vi "HV Onstate Single.vi"(8 "On/Off":string(combo), 11 "Channel":string) -> (3 "standard output":string)   [LabVIEW 2018, in "HV QMH.lvlib"]
uses:
  HV QMH.lvlib
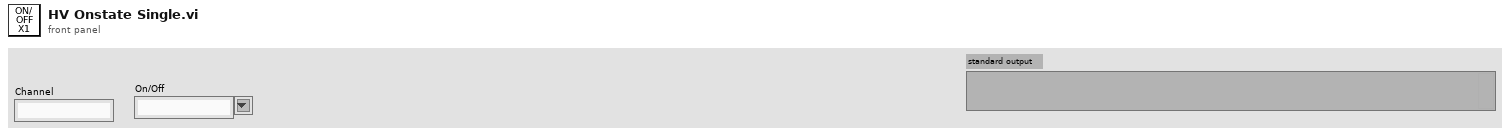
[diagram p1: front panel]
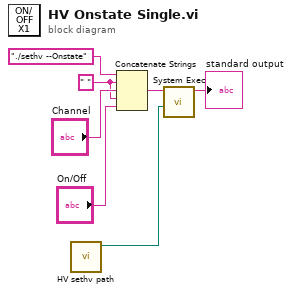
[diagram p0: block diagram]
diagram:
  w4 = " " ("string")
  n1 = call "HV sethv path.vi"() -> ("sethv filepath"=w1:path)  [unwired: 11 in]
  n2 = Concatenate Strings("./sethv --Onstate" ("string"), w4, "Channel", w4, "On/Off") -> (w7:string)
  n3 = call <vilib>:"System Exec.vi"("working directory"=w1, "command line"=w7) -> ("standard output"=→"standard output":string)  [unwired: 6 in, 3 out]
